vi "SetTemp.vi"(8 "error in (no error)":errorcluster, 9 "Humid":dbl, 10 "Temp":dbl, 11 "TempChamber Sim in":refnum<class "TempChamber Sim.lvclass">) -> (0 "error out":errorcluster, 2 "Fb":string, 3 "TempChamber Sim out":refnum<class "TempChamber Sim.lvclass">)   [LabVIEW 2018, in "QMH_Class.lvlib" / "Device.lvlib" / "TempChamber Sim.lvclass"]
uses:
  TempChamber Sim.lvclass
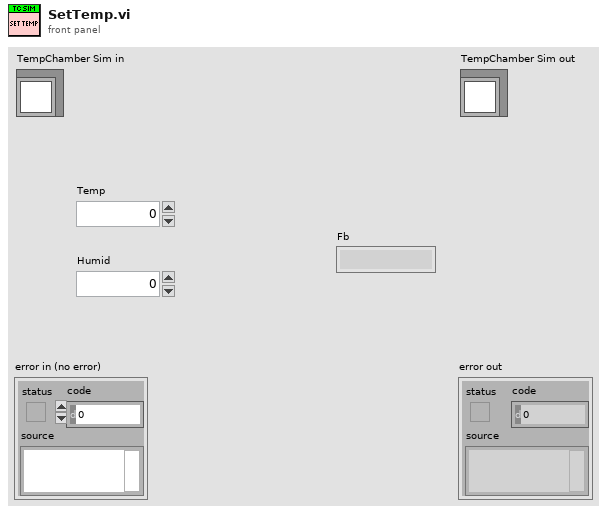
[diagram p1: front panel]
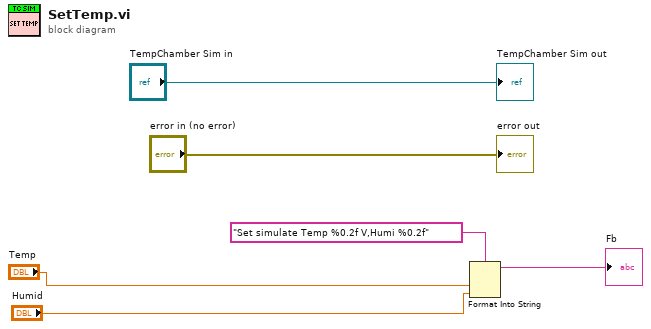
[diagram p0: block diagram]
diagram:
  n1 = Format Into String(format string="Set simulate Temp %0.2f V,Humi %0.2f", "Temp", "Humid") -> (resulting string=→"Fb":string)  [unwired: 2 in, 1 out]
  "error out" <- "error in (no error)"
  "TempChamber Sim out" <- "TempChamber Sim in"
